vi "NIRFSG_SetGeneratorMode.vi"(8 "error in (no error)":errorcluster, 10 "Gen Mode":i32(ring)=1000 items=["CW"=1000, "Arb Waveform"=1001, "Script"=1002], 11 "RFSG Handle":refnum<k15>) -> (0 "error out":errorcluster)   [LabVIEW 2015]
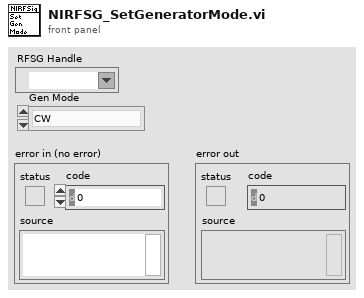
[diagram p1: front panel]
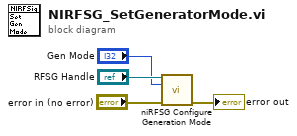
[diagram p0: block diagram]
diagram:
  n1 = call <instrlib>:"niRFSG Configure Generation Mode.vi"("instrument handle"="RFSG Handle", "generation mode"="Gen Mode", "error in"="error in (no error)") -> ("error out"=→"error out":errorcluster)  [unwired: 11 in, 1 out]
